vi "Initialize kinect systems Dani.vi"(4 "Video Format":T1, 6 "Video Res":T2, 7 "Depth Format":T3(ring)=enum."FREENECT_DEPTH_10BIT", 8 "error in (no error)":errorcluster, 9 "Led Option":T4, 10 "tilt degree":i32) -> (0 "error out":errorcluster)   [LabVIEW 2015]
uses:
  Controls/Led Control.ctl
  Controls/Video Resolution Control.ctl
  Controls/Video Format Control.ctl
  TypeDefs Host/Handle Enum.ctl
  Controls/Log Level Control.ctl
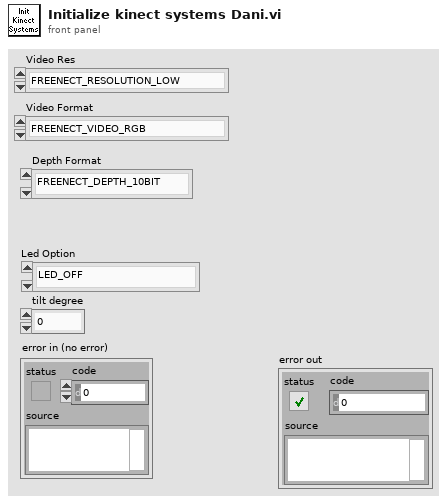
[diagram p1: front panel]
types:
  T1 = typedef "Video Format Control.ctl" = enum32{"FREENECT_VIDEO_RGB", "FREENECT_VIDEO_BAYER", "FREENECT_VIDEO_IR_8BIT", "FREENECT_VIDEO_IR_10BIT", "FREENECT_VIDEO_IR_10BIT_PACKED", "FREENECT_VIDEO_YUV_RGB", "FREENECT_VIDEO_YUV_RAW"}
  T2 = typedef "Video Resolution Control.ctl" = enum32{"FREENECT_RESOLUTION_LOW", "FREENECT_RESOLUTION_MEDIUM", "FREENECT_RESOLUTION_HIGH"}
  T3 = enum32{"FREENECT_DEPTH_11BIT", "FREENECT_DEPTH_10BIT", "FREENECT_DEPTH_11BIT_PACKED", "FREENECT_DEPTH_10BIT_PACKED", "FREENECT_DEPTH_REGISTERED", "FREENECT_DEPTH_MM"}
  T4 = typedef "Led Control.ctl" = enum32{"LED_OFF", "LED_GREEN", "LED_RED", "LED_YELLOW", "LED_BLINK_GREEN", "LED_BLINK_GREEN2", "LED_BLINK_RED_YELLOW"}
  T5 = typedef "Handle Enum.ctl" = enum16{"Set Handles", "Get Handles"}
  T6 = typedef "Log Level Control.ctl" = enum32{"FREENECT_LOG_FATAL", "FREENECT_LOG_ERROR", "FREENECT_LOG_WARNING", "FREENECT_LOG_NOTICE", "FREENECT_LOG_INFO", "FREENECT_LOG_DEBUG", "FREENECT_LOG_SPEW", "FREENECT_LOG_FLOOD"}
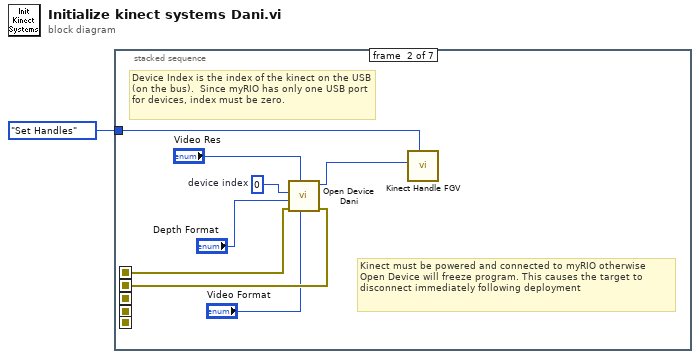
[diagram p0: block diagram]
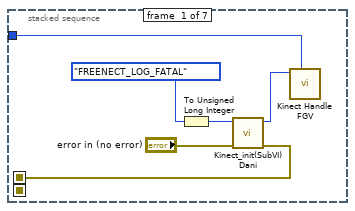
[diagram p2: hidden frame]
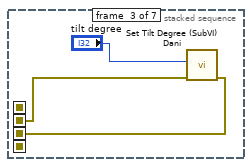
[diagram p3: hidden frame]
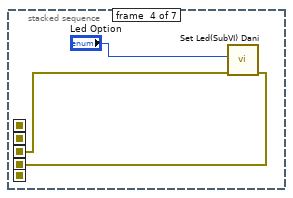
[diagram p4: hidden frame]
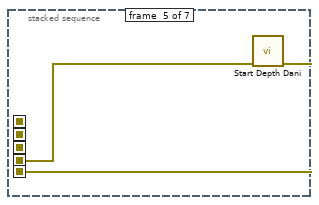
[diagram p5: hidden frame]
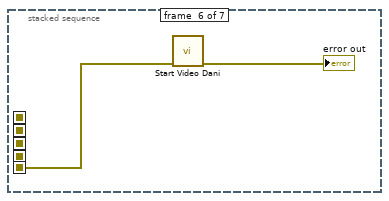
[diagram p6: hidden frame]
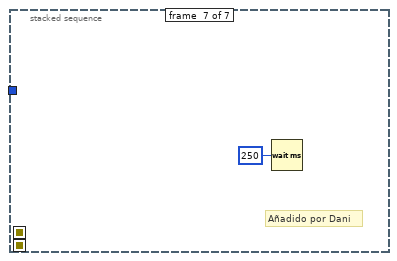
[diagram p7: hidden frame]
diagram:
  n1 = stacked-sequence {
    seq-local: [w4 _ _ _ _ _ _] -> [_ w14 _ _ _ _ _]
    seq-local: [_ w13 _ _ _ _ _] -> [_ _ w17 _ _ _ _]
    seq-local: [_ _ w16 _ _ _ _] -> [_ _ _ w20 _ _ _]
    seq-local: [_ _ _ w19 _ _ _] -> [_ _ _ _ w23 _ _]
    seq-local: [_ _ _ _ w22 _ _] -> [_ _ _ _ _ w25 _]
    tunnel: Handle_Enum."Set Handles" ("Handle Command") -> [w3 w11 _ _ _ _ _]
    frame #0 {
      n2 = To Unsigned Long Integer(number=Log_Level_Control."FREENECT_LOG_FATAL" ("Log Level")) -> (unsigned 32bit integer=w7:u32)
      n3 = call "Kinect_init(SubVI) Dani.vi"("error in (no error)"="error in (no error)", "log_level"=w7) -> ("error out"=w4:errorcluster, "Context_handle"=w2:i64)  [unwired: 8 in]
      n4 = call "Kinect Handle FGV.vi"("Handle Command"=w3, "Kinect Handle In"=w2) -> ()  [unwired: 8 in, 2 out]
    }
    frame #1 {
      w12 = 0  # device index
      # "Device Index is the index of the kinect on the USB (on the bus).  Since myRIO has only one USB port for devices, index must be zero."
      # "Kinect must be powered and connected to myRIO otherwise Open Device will freeze program. This causes the target to disconnect immediately following deployment"
      n5 = call "Open Device Dani.vi"("Video Format"="Video Format", "Video Res"="Video Res", "error in (no error)"=w14, "Depth Format"="Depth Format", "device index"=w12) -> ("error out"=w13:errorcluster, "handle"=w10:i64)  [unwired: 5 in]
      n6 = call "Kinect Handle FGV.vi"("Handle Command"=w11, "Context Handle In"=w10) -> ()  [unwired: 8 in, 2 out]
    }
    frame #2 {
      n7 = call "Set Tilt Degree (SubVI) Dani.vi"("degree"="tilt degree", "error in (no error)"=w17) -> ("error out"=w16:errorcluster)  [unwired: 8 in]
    }
    frame #3 {
      n8 = call "Set Led(SubVI) Dani.vi"("error in (no error)"=w20, "Led Option"="Led Option") -> ("error out"=w19:errorcluster)  [unwired: 9 in]
    }
    frame #4 {
      n9 = call "Start Depth Dani.vi"("error in (no error)"=w23) -> ("error out"=w22:errorcluster)  [unwired: 10 in]
    }
    frame #5 {
      n10 = call "Start Video Dani.vi"("error in (no error)"=w25) -> ("error out"=→"error out":errorcluster)  [unwired: 10 in]
    }
    frame #6 {
      # "Añadido por Dani"
      n11 = Wait (ms)(milliseconds to wait=u32 250) -> ()  [unwired: 1 out]
    }
  }
